vi "AQT_set_connection.vi"(9 "data":u32, 10 "address":u32, 11 "hnd":u32) -> (2 "return codes":u32[](array[numeric]), 3 "hnd out":u32)   [LabVIEW 2012]
uses:
  <userlib>/okFrontPanel/okFrontPanel.lvlib
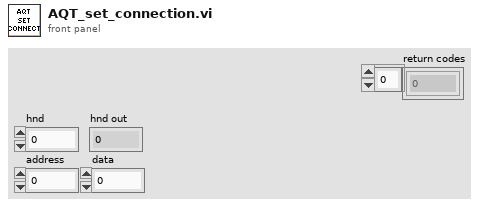
[diagram p1: front panel]
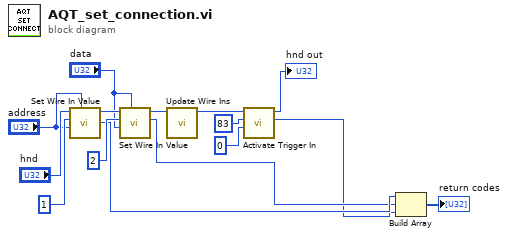
[diagram p0: block diagram]
diagram:
  n1 = call <userlib>:"Set Wire In Value.vi"("mask"="address", "val"="address", "ep"=1, "hnd"="hnd") -> ("function return"=w4:u32, "hnd out"=w9:u32)  [unwired: 6 in]
  n2 = call <userlib>:"Set Wire In Value.vi"("mask"="data", "val"="data", "ep"=2, "hnd"=w9) -> ("function return"=w3:u32, "hnd out"=w10:u32)  [unwired: 6 in]
  n3 = call <userlib>:"Update Wire Ins.vi"("hnd"=w10) -> ("hnd out"=w11:u32)  [unwired: 10 in]
  n4 = call <userlib>:"Activate Trigger In.vi"("bit"=0, "epAddr"=83, "hnd"=w11) -> ("function return"=w2:u32, "hnd out"=→"hnd out":u32)  [unwired: 7 in]
  n5 = Build Array(w4, w3, w2) -> (→"return codes":u32[])
